vi "testAll.vi"(8 "error in (no error)":errorcluster) -> (0 "error out":errorcluster)   [LabVIEW 2018]
doc: "Run all the unit tests."
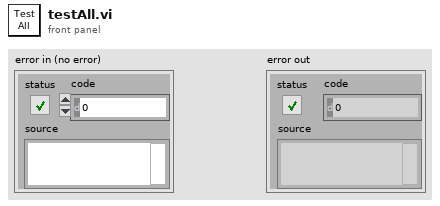
[diagram p1: front panel]
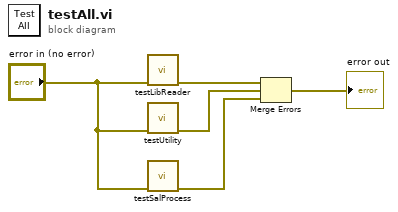
[diagram p0: block diagram]
diagram:
  n1 = call "testLibReader.vi"("error in (no error)"="error in (no error)") -> ("error out"=w5:errorcluster)  [unwired: 10 in]
  n2 = call "testUtility.vi"("error in (no error)"="error in (no error)") -> ("error out"=w4:errorcluster)  [unwired: 10 in]
  n3 = call "testSalProcess.vi"("error in (no error)"="error in (no error)") -> ("error out"=w1:errorcluster)  [unwired: 10 in]
  n4 = Merge Errors(w5, w4, w1) -> (→"error out":errorcluster)
